vi "CR-导丝颗粒检测1.vi"(8 "error in (no error)":errorcluster caption="错误输入（无错误）", 11 "名称或相对路径":string="Template Program") -> (0 "error in (no error) 2":errorcluster caption="错误输入（无错误）")   [LabVIEW 2017]
uses:
  Picture/SaveButtom.ctl
  Global System.vi
  <vilib>/Utility/xml.llb/Write to XML File(string).vi
panel:
  in  "获取图像":bool
  in  "ROI获取":bool
  in  "创建模板":bool
  in  "保存图像":bool
  out "添加的路径":path
  in  "刷新":bool
  in  "测试按钮":bool
  in  "保存按钮":bool
  in  "Main":enum32{"主参数", "颜色模板匹配参数 ", "测试效果"}(tab)
  in  "导丝颗粒物检测1基础参数":T1={"IsNorImage"=TRUE, "Exposure Values"=100289, "ImagePath"=path "C:/Users/hedongpo/Desktop/514-hdp/Alignment Assemble System/Test Picture/B/3.bmp"} caption="参数界面" {"Exposure Values" scale=0.0..200000.0}
  in  "导丝颗粒物检测1参数":T3={"Rectangle"={"Left"=0, "Top"=0, "Right"=0, "Bottom"=0, "Rotation"=0.0}, "Match Mode "=0, "Minimum Match Score "=800.0, "Number of Matches Requested"=1, "Color Sensitivity "=0, "Color Score Weight "=500.0, "Search Strategy "=0, "Subpixel Accuracy "=FALSE, "Rotation Angle Ranges (degrees)"=[{"Min"=-180.0, "Max"=180.0}], "Match Offset"={"X"=0.0, "Y"=0.0}, "模板路径"=path "C:/Users/delluser001/Desktop/PowerLine Inspect System/Source Code/Template Program/potteryTemplete/Color.png"} {"Search Strategy" items=["Conservative", "Balance", "Aggressive", "Very Aggressive"]; "Color Sensitivity" items=["Low Sensitivity", "Medium Sensitivity", "High Sensitivity"]; "Match Mode" items=["Shift Invariant", "Rotation Invariant"]; "Rectangle"."Rotation" format="%.2f"; "Rectangle"."Left" scale=0.0..1024.0; "Rectangle"."Right" scale=0.0..1024.0}
  out "Number of Features Found":i32
  out "颗粒物有无显示":bool
  in  "Feature Points Strength":string[][](table)
  out "原始图像":T4(plugin-control)
  out "路径输出":path
  in  "Vision Paramter Save Buttom":T5
  out "system time":string
  in  "取消按钮":bool
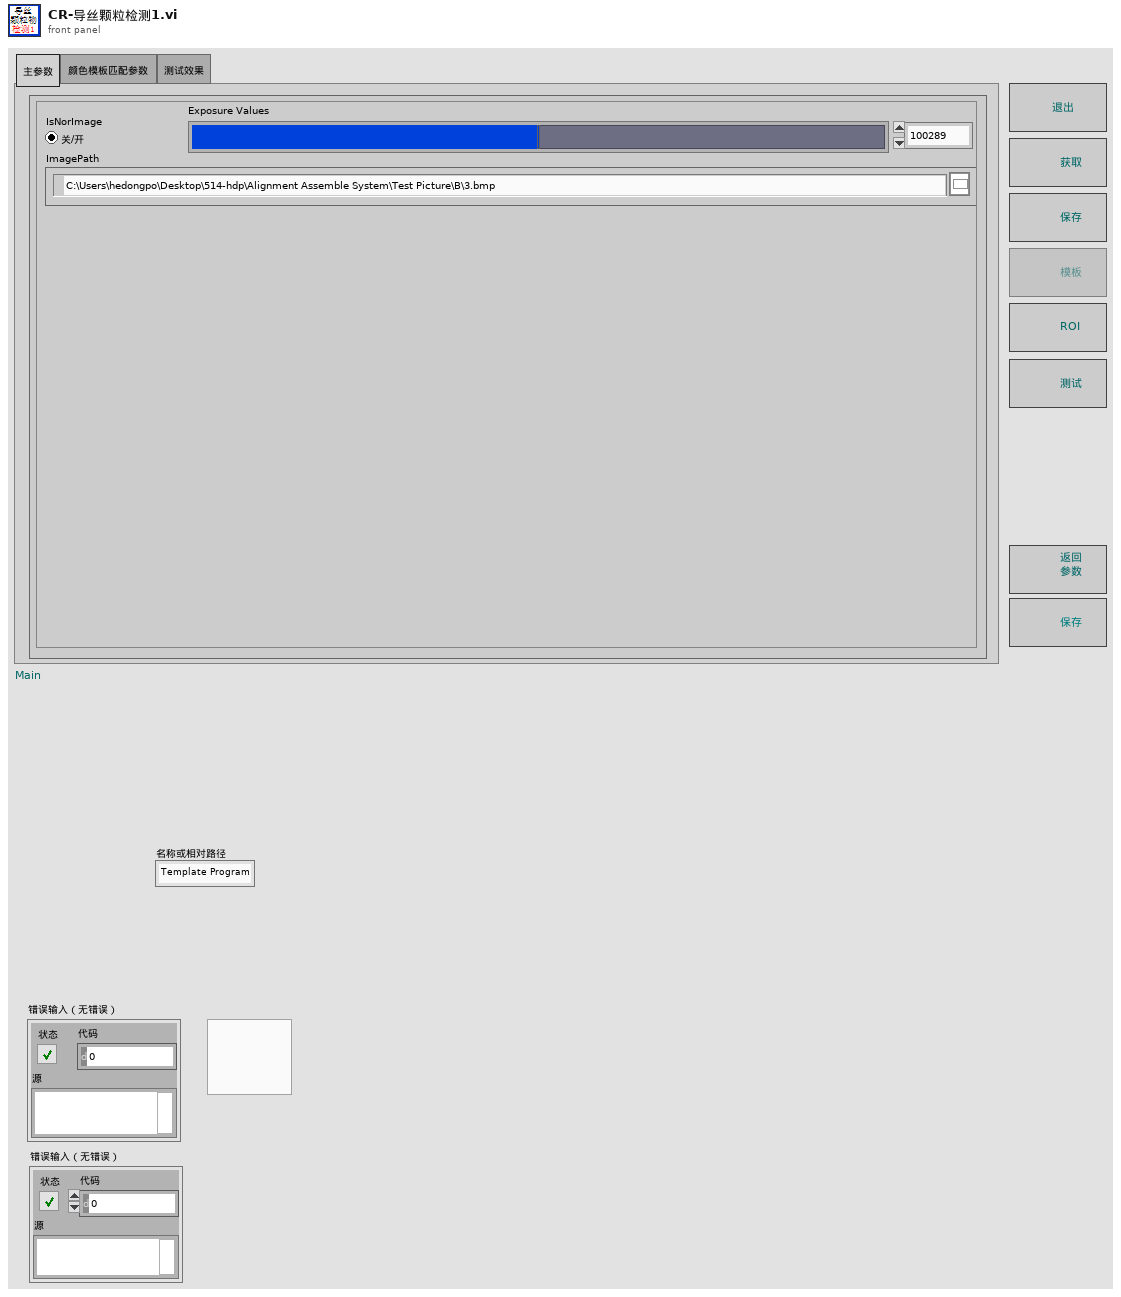
[diagram p1: front panel]
types:
  T1 = cluster{"IsNorImage":bool, "Exposure Values":u32, "ImagePath":path}
  T2 = typedef "IMAQ Rectangle" = cluster{"Left":i32, "Top":i32, "Right":i32, "Bottom":i32, "Rotation":dbl}
  T3 = cluster{"Rectangle":T2, "Match Mode ":u32, "Minimum Match Score ":sgl, "Number of Matches Requested":i32, "Color Sensitivity ":u32, "Color Score Weight ":sgl, "Search Strategy ":u32, "Subpixel Accuracy ":bool, "Rotation Angle Ranges (degrees)":cluster{"Min":sgl, "Max":sgl}[], "Match Offset":cluster{"X":sgl, "Y":sgl}, "模板路径":path}
  T4 = typedef "IMAQ Image.ctl" = refnum<image>
  T5 = typedef "SaveButtom.ctl" = bool
  T6 = cluster{"index":i32, "this vi":refnum<vi>, "error out":errorcluster}
  T7 = cluster{"master data":string, "priority":u16, "secondary data":string[]}
  T8 = cluster{"case name":string[], "queue array":refnum<queue>[]}
  T9 = cluster{"Global Rectangle":i32[], "Contours":cluster{"Contour Type":u32, "ROI Type":u32, "Points":i32[]}[]}
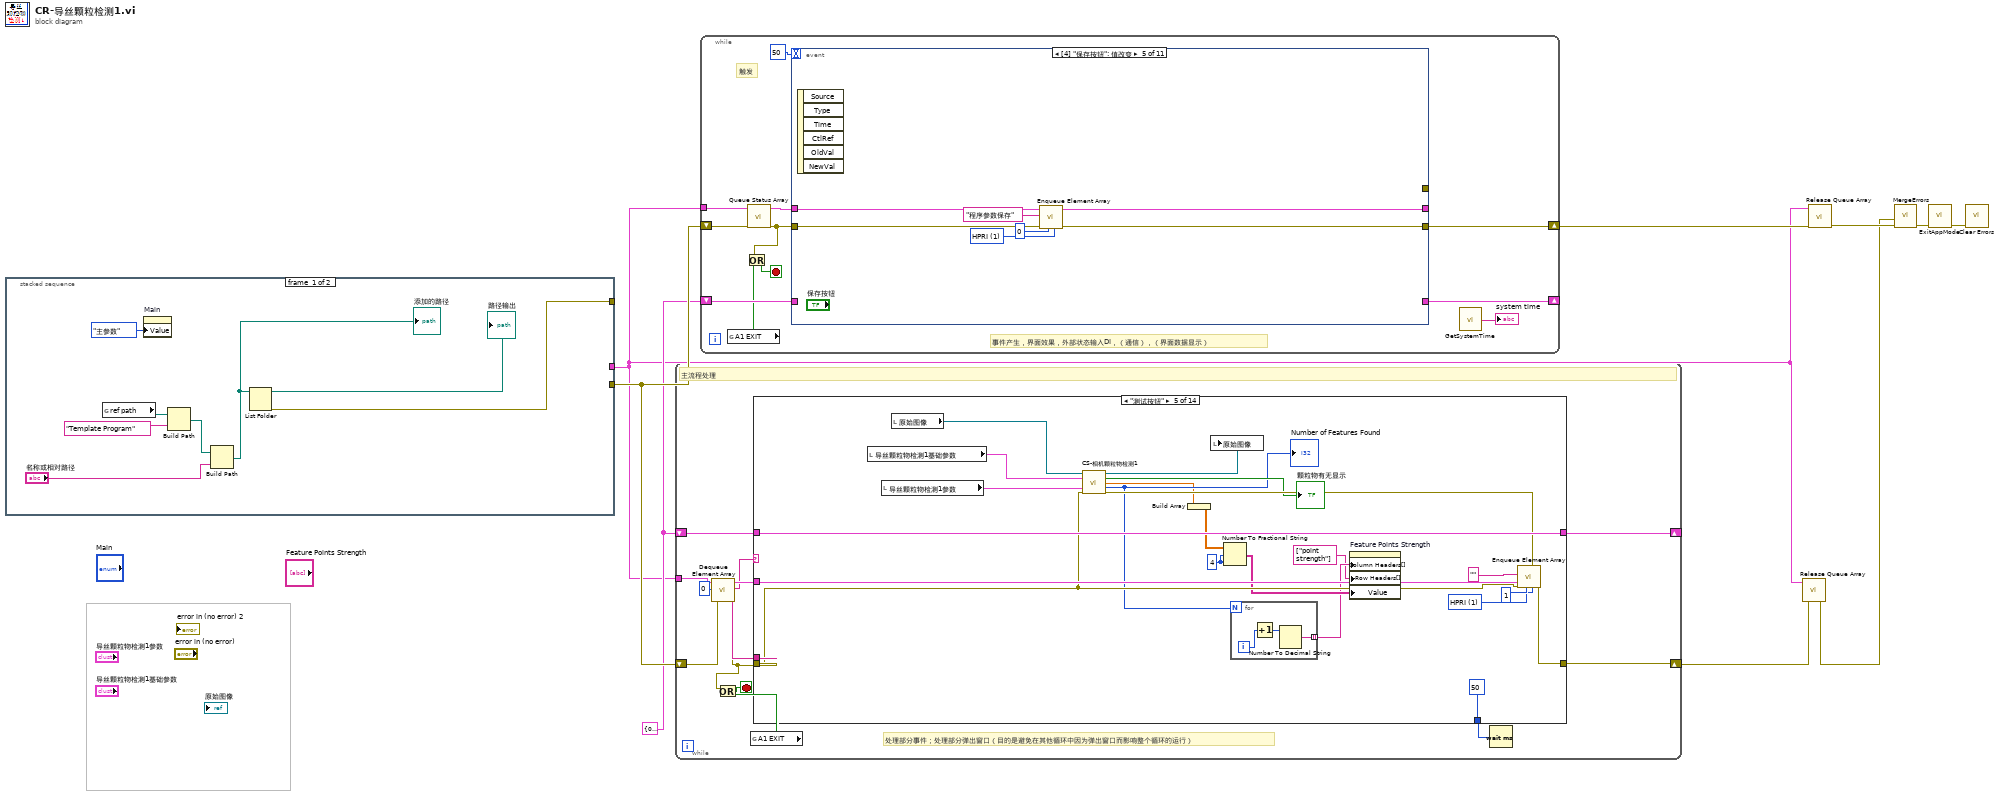
[diagram p0: block diagram]
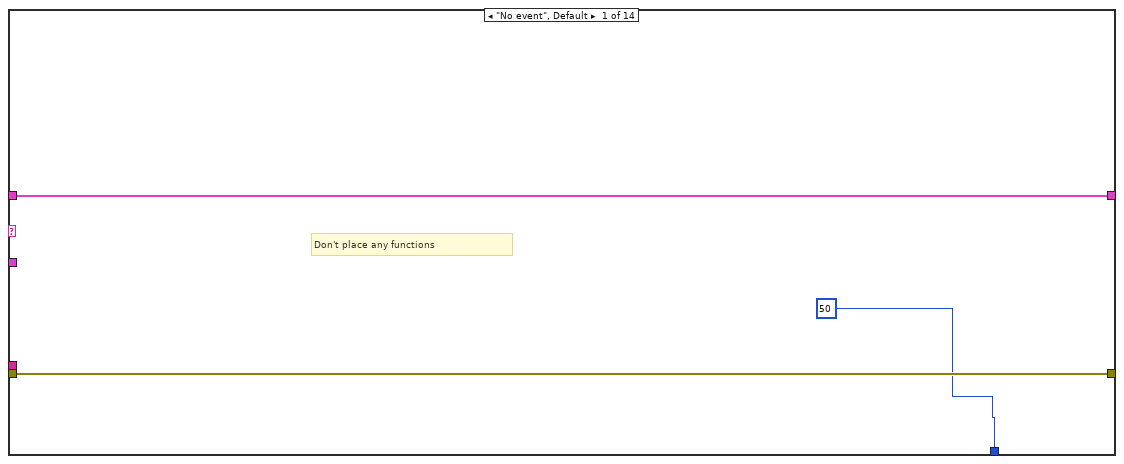
[diagram p2: hidden frame]
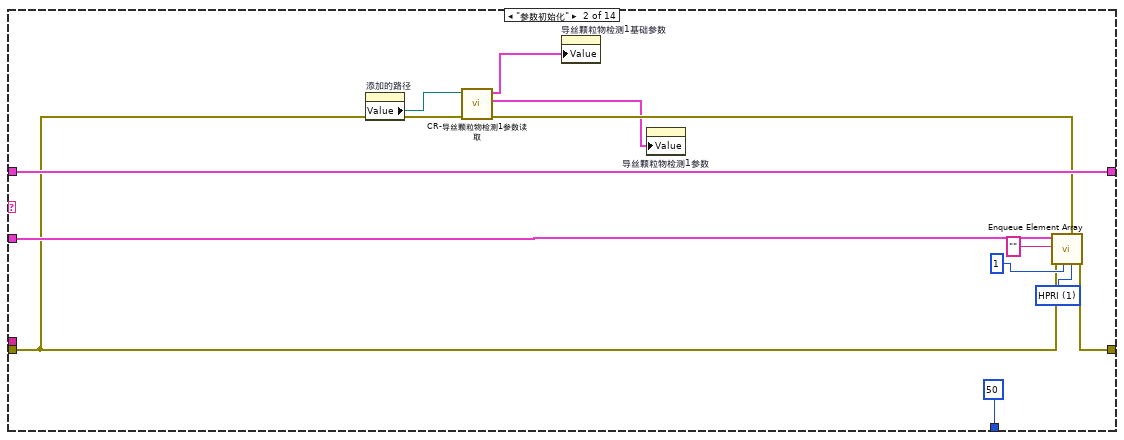
[diagram p3: hidden frame]
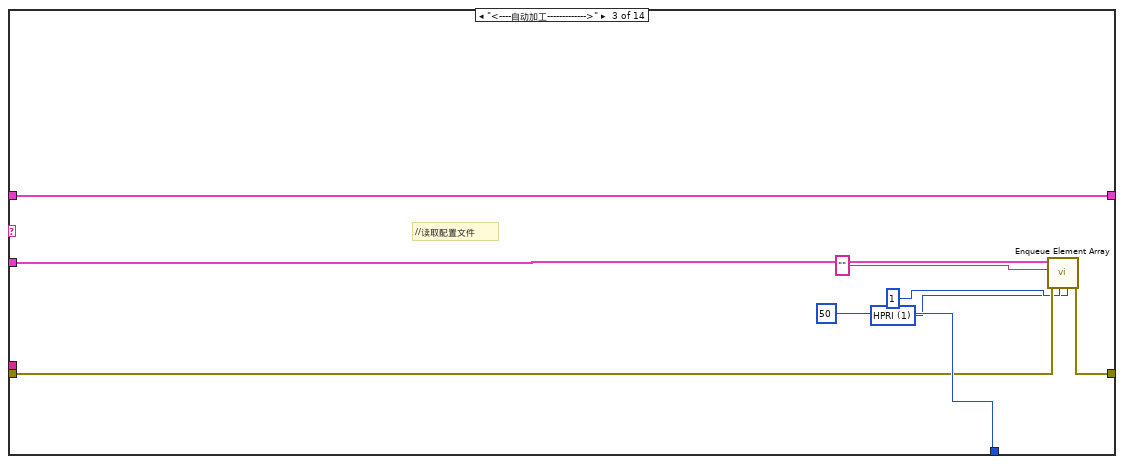
[diagram p4: hidden frame]
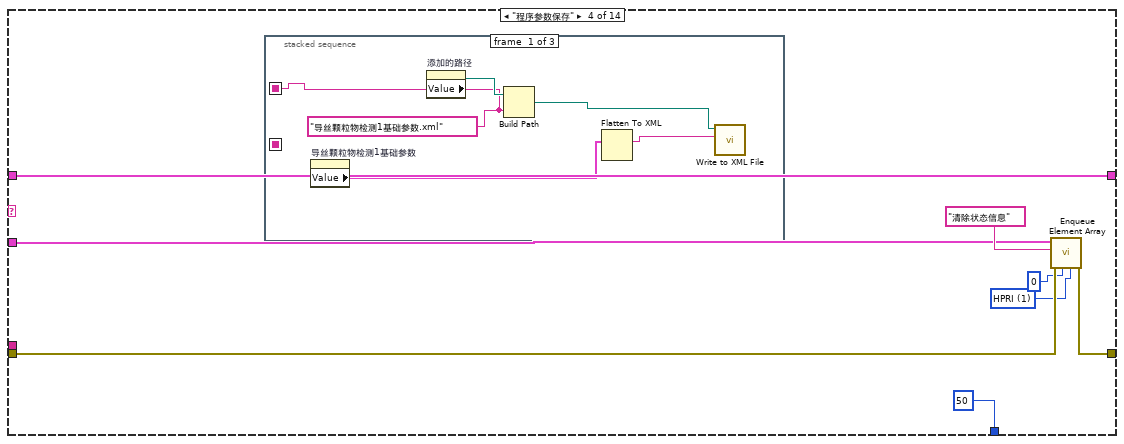
[diagram p5: hidden frame]
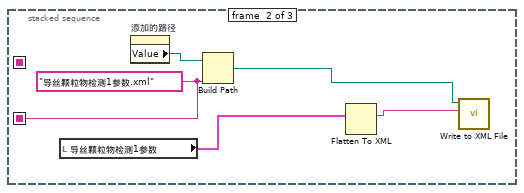
[diagram p6: hidden frame]
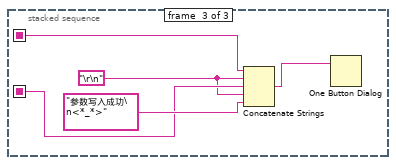
[diagram p7: hidden frame]
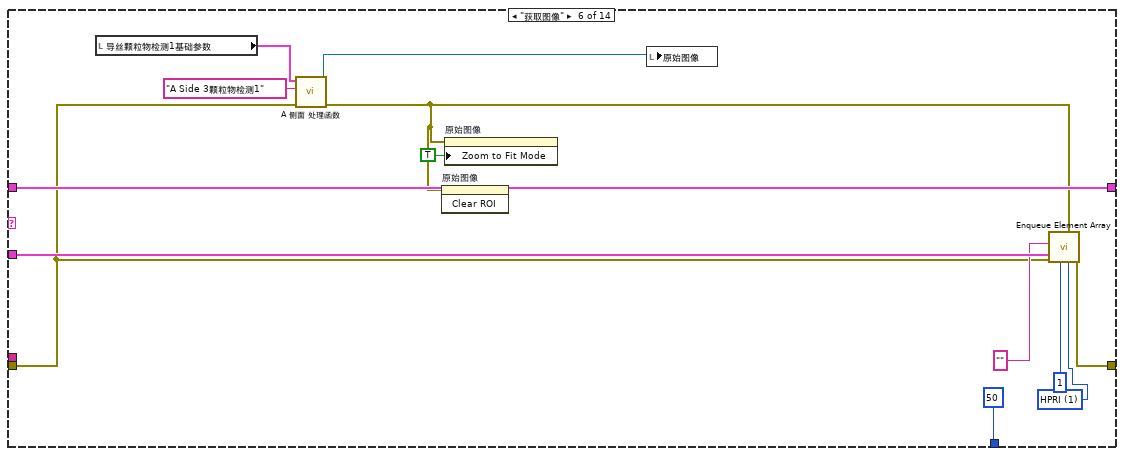
[diagram p8: hidden frame]
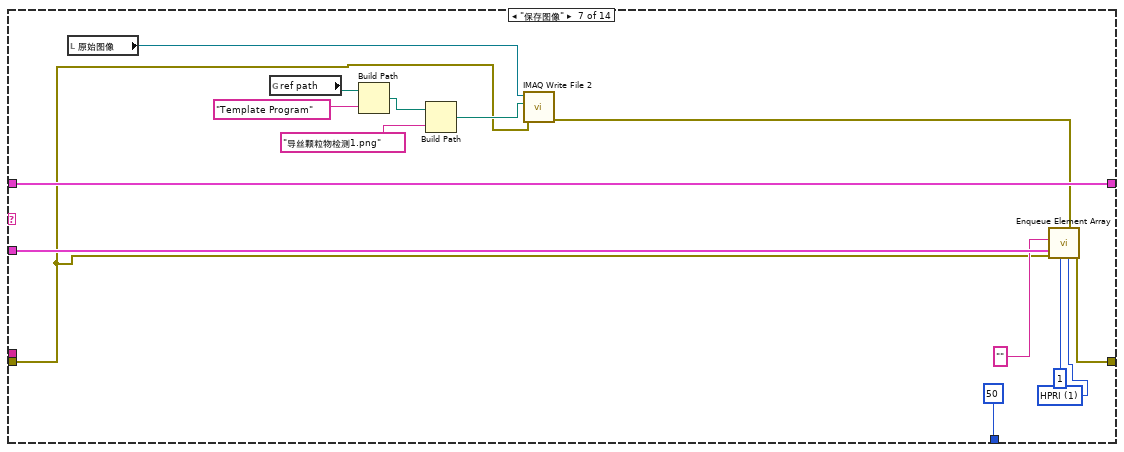
[diagram p9: hidden frame]
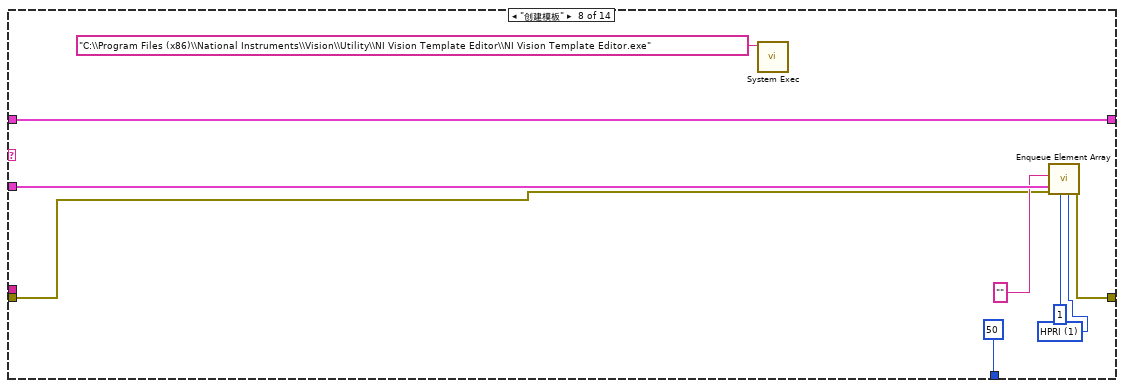
[diagram p10: hidden frame]
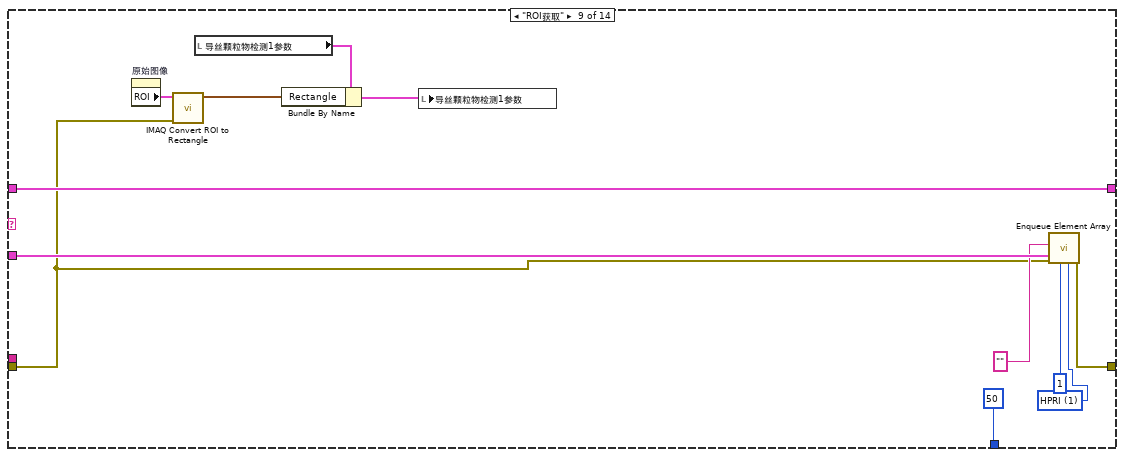
[diagram p11: hidden frame]
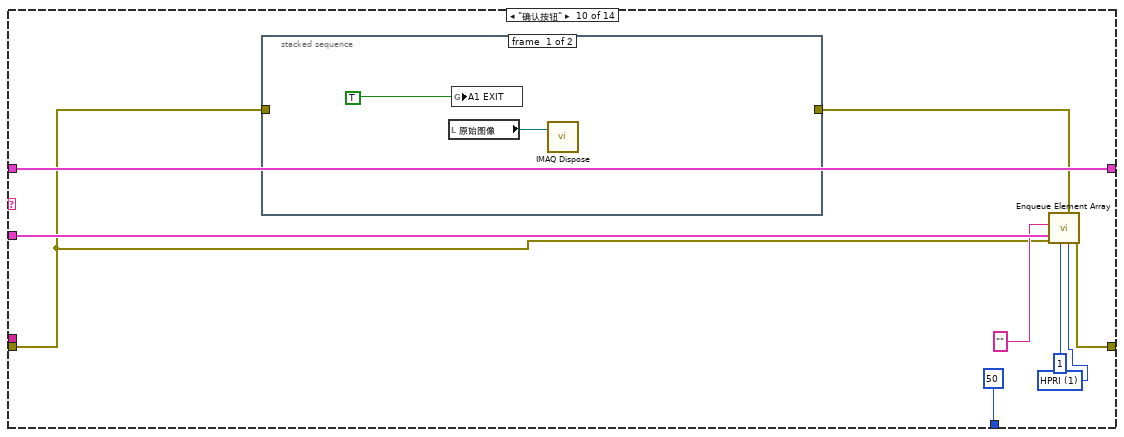
[diagram p12: hidden frame]
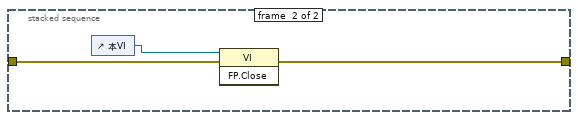
[diagram p13: hidden frame]
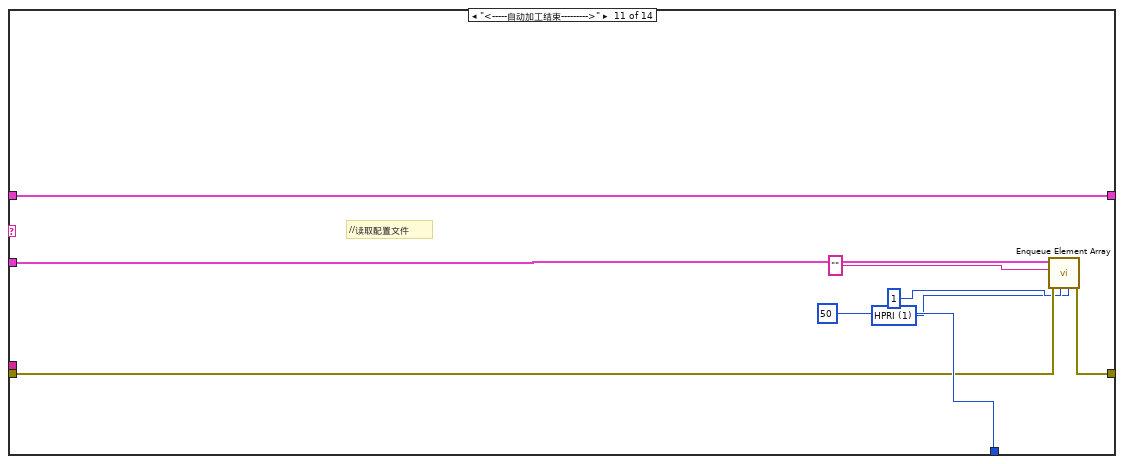
[diagram p14: hidden frame]
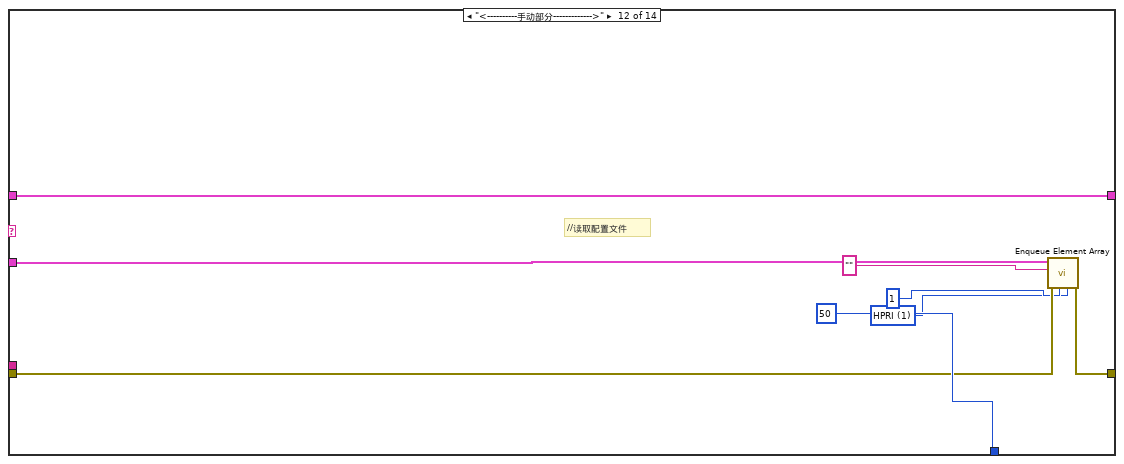
[diagram p15: hidden frame]
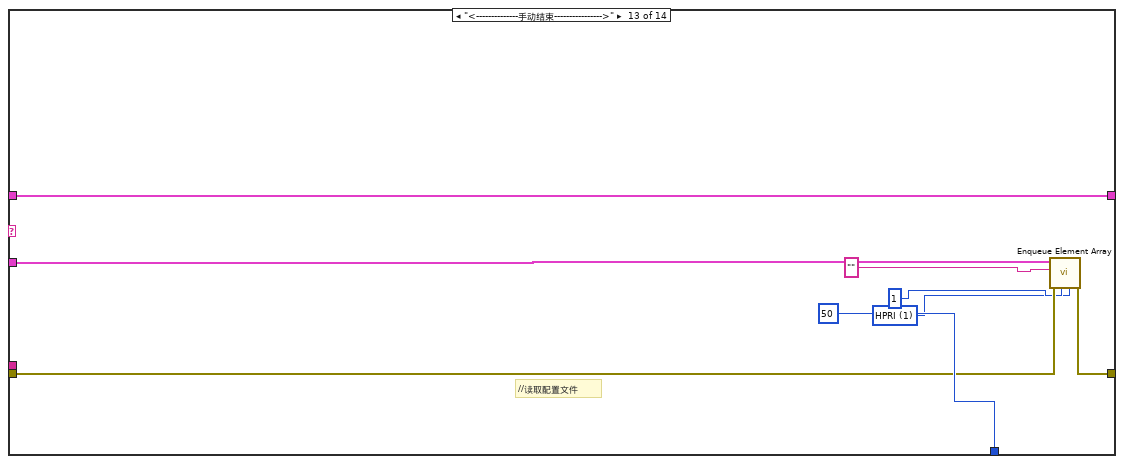
[diagram p16: hidden frame]
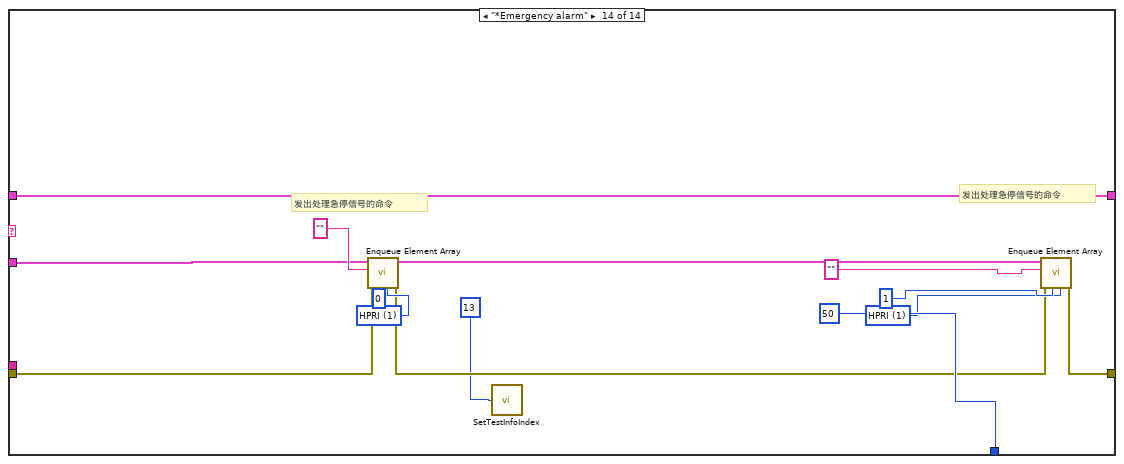
[diagram p17: hidden frame]
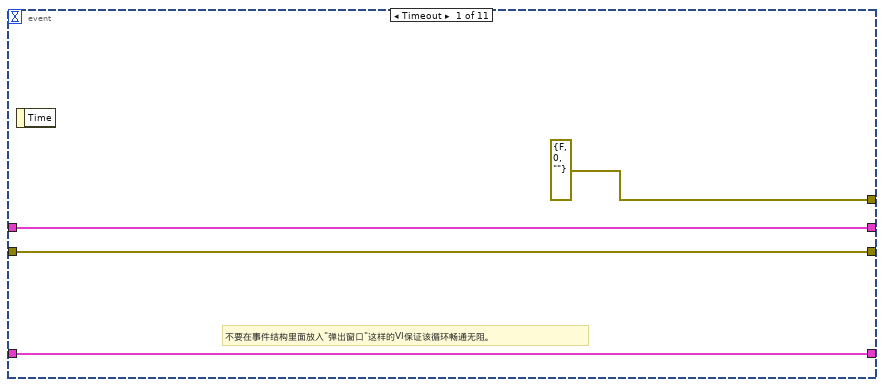
[diagram p18: hidden frame]
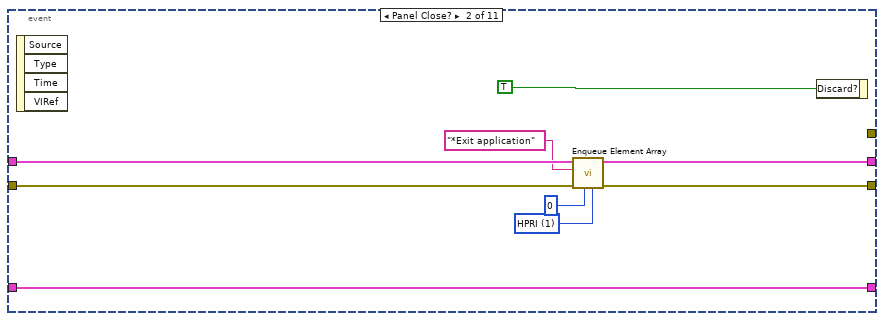
[diagram p19: hidden frame]
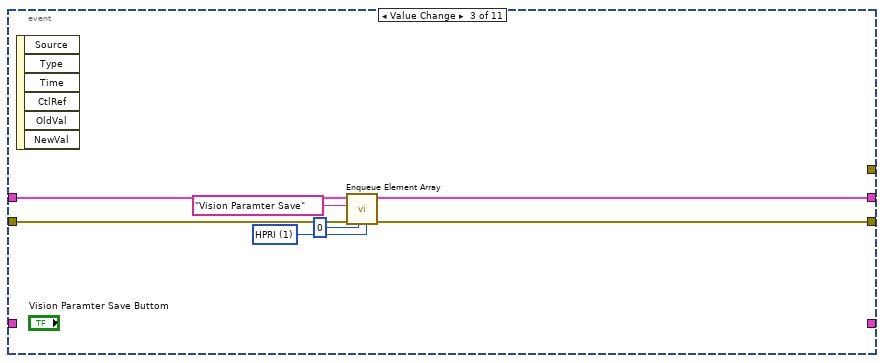
[diagram p20: hidden frame]
diagram:
  w4 = T6 {"index"=0, "this vi"=refnum, "error out"={"status"=FALSE, "code"=0, "source"=""}} ("parameter buffer")
  n1 = stacked-sequence {
    tunnel: [w16 _] -> _
    tunnel: [_ w19] -> w5
    tunnel: [_ w18] -> w1
    frame #0 {
      n2 = global read "Global System.vi" "ref path"() -> (w14:path)
      n3 = property on="Main" class="TabCtl (严格)"("Value"=enum32{"主参数", "颜色模板匹配参数 ", "测试效果"}."主参数" ("Main")) -> ()  [unwired: 2 in, 2 out]
      n4 = Build Path(base path=w14, name or relative path="Template Program" ("名称或相对路径")) -> (appended path=w12:path)
      n5 = Build Path(base path=w12, name or relative path="名称或相对路径") -> (appended path=w10:path)
      "添加的路径" <- w10
      n6 = List Folder(path=w10) -> (path out=→"路径输出":path, error out=w16:errorcluster)  [unwired: 3 in, 2 out]
    }
    frame #1 {
      w27 = string[] ["comm queue1", "data queue 11", "data queue 12", "data queue 13", "data queue 14"]  # queue name
      w28 = 4  # queue num
      w29 = T7 {"master data"="", "priority"=0, "secondary data"=[]}  # element data type
      n7 = call "Obtain Queue Array.vi"("queue name"=w27, "element data type"=w29, "queue num"=w28) -> ("error out"=w23:errorcluster, "queue out"=w24:T8)  [unwired: 2 in, 1 out]
      n8 = call "Enqueue Element Array.vi"("queue index"=0, "error in"=w23, "master data"="参数初始化", "queue in"=w24) -> ("error out"=w22:errorcluster, "queue out"=w21:T8)  [unwired: 6 in]
      n9 = disable-structure shown="启用" {
        disable-tunnel: w22 -> [w35 w36]
        disable-tunnel: w21 -> [w34 w37]
        disable-tunnel: "Loading Variable" ("master data") -> [w33 _]
        disable-tunnel: [w31 w36] -> w19
        disable-tunnel: [w30 w37] -> w18
        frame Disabled {
          n10 = call "Enqueue Element Array.vi"("queue index"=12, "error in"=w35, "master data"=w33, "queue in"=w34) -> ("error out"=w31:errorcluster, "queue out"=w30:T8)  [unwired: 6 in]
        }
        frame Enabled {
        }
      }
    }
  }
  n11 = while {
    shift-right: [w50] -> w3
    shift-left: w5 -> [w41]
    shift-right: [w47] -> _
    shift-left: w4 -> [w48]
    tunnel: w1 -> [w43]
    stop <- w38 stop-if-true
    # "处理部分事件；处理部分弹出窗口（目的是避免在其他循环中因为弹出窗口而影响整个循环的运行）"
    # "主流程处理"
    n12 = call "Dequeue Element Array.vi"("queue in"=w43, "queue index"=0, "error in"=w41) -> ("queue out"=w46:T8, "master data"=w45:string, "secondary data"=w44:string[], "error out"=w40:errorcluster)  [unwired: 2 in, 1 out]
    n13 = global read "Global System.vi" "A1 EXIT"() -> (w39:bool)
    n14 = Or(x=w40, y=w39) -> (x .or. y?=w38:bool)
    n15 = case shown="\"测试按钮\"" w45 {
      tunnel: w46 -> [_ w64 w72 w74 w116 w132 w147 w156 w168 w177 w190 w198 w206 w212]
      tunnel: w40 -> [w52 w57 w68 w78 w109 w123 w134 w150 w161 w171 w186 w194 w202 w209]
      tunnel: [w52 w63 w71 w80 w115 w131 w146 w155 w167 w176 w189 w197 w205 w220] -> w50
      tunnel: [50 50 50 50 50 50 50 50 50 50 50 50 50 50] -> w49
      tunnel: w48 -> [w53 w59 w69 w75 w111 w127 w142 w151 w163 w172 w187 w195 w203 w218]
      tunnel: [w53 w59 w69 w75 w111 w127 w142 w151 w163 w172 w187 w195 w203 w218] -> w47
      tunnel: w44 -> [_ _ _ _ _ _ _ _ _ _ _ _ _ _]
      frame "No event", Default {
        # "Don't place any functions"
      }
      frame "参数初始化" {
        w60 = u16 1 items=["HPRI"=1, "LPRI"=0] ("priority")
        n16 = property on="添加的路径" class="Path"() -> ("Value"=w58:path)  [unwired: 2 in, 2 out]
        n17 = call "CR-导丝颗粒物检测1参数读取.vi"("error in (no error)"=w57, "基路径"=w58) -> ("error out"=w56:errorcluster, "导丝颗粒物检测1参数"=w54:T3, "导丝颗粒物检测1基础参数"=w55:T1)  [unwired: 6 in]
        n18 = property on="导丝颗粒物检测1基础参数" class="Clust (严格)"("Value"=w55) -> ()  [unwired: 2 in, 2 out]
        n19 = property on="导丝颗粒物检测1参数" class="Clust (严格)"("Value"=w54) -> ()  [unwired: 2 in, 2 out]
        n20 = call "Enqueue Element Array.vi"("priority"=w60, "device error in"=w56, "queue index"=1, "error in"=w57, "master data"="" ("Element 1"), "queue in"=w64) -> ("error out"=w63:errorcluster)  [unwired: 4 in, 1 out]
      }
      frame "<----自动加工------------->" {
        w66 = u16 1 items=["HPRI"=1, "LPRI"=0] ("priority")
        # "//读取配置文件"
        n21 = call "Enqueue Element Array.vi"("priority"=w66, "queue index"=1, "error in"=w68, "master data"="" ("Element 1"), "queue in"=w72) -> ("error out"=w71:errorcluster)  [unwired: 5 in, 1 out]
      }
      frame "程序参数保存" {
        w76 = u16 1 items=["HPRI"=1, "LPRI"=0] ("priority")
        n22 = stacked-sequence {
          seq-local: [_ w88 _] -> [_ _ w94]
          seq-local: [w82 _ _] -> [_ _ w92]
          frame #0 {
            w82 = "导丝颗粒物检测1基础参数.xml" ("名称或相对路径")
            n23 = property on="导丝颗粒物检测1基础参数" class="Clust (严格)"() -> ("Value"=w85:T1)  [unwired: 2 in, 2 out]
            n24 = property on="添加的路径" class="Path"() -> ("Value"=w86:path)  [unwired: 2 in, 2 out]
            n25 = Build Path(base path=w86, name or relative path=w82) -> (appended path=w83:path)
            n26 = Flatten To XML(anything=w85) -> (xml string=w84:string)
            n27 = call-poly <vilib>:"Write to XML File.vi"("XML Input"=w84, "XML File Path"=w83) -> ()  [unwired: 7 in, 3 out]
          }
          frame #1 {
            w88 = "导丝颗粒物检测1参数.xml" ("名称或相对路径")
            n28 = local read "导丝颗粒物检测1参数"() -> (w87:T3)
            n29 = property on="添加的路径" class="Path"() -> ("Value"=w91:path)  [unwired: 2 in, 2 out]
            n30 = Build Path(base path=w91, name or relative path=w88) -> (appended path=w89:path)
            n31 = Flatten To XML(anything=w87) -> (xml string=w90:string)
            n32 = call-poly <vilib>:"Write to XML File.vi"("XML Input"=w90, "XML File Path"=w89) -> ()  [unwired: 7 in, 3 out]
          }
          frame #2 {
            w93 = "\r\n"
            n33 = Concatenate Strings(w92, w93, w94, w93, "参数写入成功\n<*_*>" ("消息")) -> (w95:string)
            n34 = One Button Dialog(message=w95) -> ()  [unwired: 1 in, 1 out]
          }
        }
        n35 = call "Enqueue Element Array.vi"("priority"=w76, "queue index"=0, "error in"=w78, "master data"="清除状态信息" ("Element 1"), "queue in"=w74) -> ("error out"=w80:errorcluster)  [unwired: 5 in, 1 out]
      }
      frame "测试按钮" {
        w101 = i16 4 ("精度(6)")
        w112 = u16 1 items=["HPRI"=1, "LPRI"=0] ("priority")
        n36 = local read "导丝颗粒物检测1基础参数"() -> (w110:T1)
        n37 = local read "导丝颗粒物检测1参数"() -> (w105:T3)
        n38 = local read "原始图像"() -> (w107:T4)
        n39 = call "CS-相机颗粒物检测1.vi"("Image in"=w107, "相机颗粒物检测1基础参数"=w110, "相机颗粒物检测1参数"=w105, "error in (no error)"=w109) -> ("Image out"=w108:T4, "颗粒物有无显示"=→"颗粒物有无显示":bool, "颗粒物大小显示"=w102:dbl[], "Number of Features Found"=w103:i32, "error out"=w106:errorcluster)  [unwired: 6 in, 1 out]
        "Number of Features Found" <- w103
        n40 = Build Array(w102) -> (w100:dbl[][])
        n41 = local write "原始图像"(w108) -> ()
        n42 = Number To Fractional String(number=w100, width (-)=w101, precision (6)=w101) -> (F-format string=w99:string[][])  [unwired: 1 in]
        n43 = for {
          N: w103 -> [_]
          tunnel: [w118] -> w98 mode=indexing
          i -> [w120]
          n44 = Increment(x=w120) -> (x+1=w119:i32)
          n45 = Number To Decimal String(number=w119) -> (decimal integer string=w118:string)  [unwired: 1 in]
        }
        n46 = property on="Feature Points Strength" class="Tbl (严格)"("Column Headers[]"=w98, "Row Headers[]"=string[] ["point strength"] ("列首字符串[]"), "Value"=w99) -> ()  [unwired: 2 in, 2 out]
        n47 = call "Enqueue Element Array.vi"("priority"=w112, "device error in"=w106, "queue index"=1, "error in"=w109, "master data"="" ("Element 1"), "queue in"=w116) -> ("error out"=w115:errorcluster)  [unwired: 4 in, 1 out]
      }
      frame "获取图像" {
        w128 = u16 1 items=["HPRI"=1, "LPRI"=0] ("priority")
        n48 = local read "导丝颗粒物检测1基础参数"() -> (w125:T1)
        n49 = call "A 侧面 处理函数.vi"("error in (no error)"=w123, "Image Name"="A Side 3颗粒物检测1", "ParamsUI"=w125) -> ("error out"=w121:errorcluster, "Image out"=w124:T4)  [unwired: 5 in, 2 out]
        n50 = invoke on="原始图像" class="ImageControl" method="Clear ROI"(error in=w121) -> ()  [unwired: 2 in, 3 out]
        n51 = property on="原始图像" class="ImageControl"(error in=w121, "Zoom to Fit Mode"=TRUE) -> ()  [unwired: 1 in, 2 out]
        n52 = local write "原始图像"(w124) -> ()
        n53 = call "Enqueue Element Array.vi"("priority"=w128, "device error in"=w121, "queue index"=1, "error in"=w123, "master data"="" ("Element 1"), "queue in"=w132) -> ("error out"=w131:errorcluster)  [unwired: 4 in, 1 out]
      }
      frame "保存图像" {
        w143 = u16 1 items=["HPRI"=1, "LPRI"=0] ("priority")
        n54 = local read "原始图像"() -> (w135:T4)
        n55 = global read "Global System.vi" "ref path"() -> (w141:path)
        n56 = Build Path(base path=w141, name or relative path="Template Program" ("名称或相对路径")) -> (appended path=w139:path)
        n57 = Build Path(base path=w139, name or relative path="导丝颗粒物检测1.png" ("名称或相对路径")) -> (appended path=w137:path)
        n58 = call-poly "IMAQ Write File 2"("error in (no error)"=w134, "File Path"=w137, "Image"=w135) -> ("error out"=w136:errorcluster)  [unwired: 7 in, 1 out]
        n59 = call "Enqueue Element Array.vi"("priority"=w143, "device error in"=w136, "queue index"=1, "error in"=w134, "master data"="" ("Element 1"), "queue in"=w147) -> ("error out"=w146:errorcluster)  [unwired: 4 in, 1 out]
      }
      frame "创建模板" {
        w152 = u16 1 items=["HPRI"=1, "LPRI"=0] ("priority")
        n60 = call <vilib>:"System Exec.vi"("command line"="C:\\Program Files (x86)\\National Instruments\\Vision\\Utility\\NI Vision Template Editor\\NI Vision Template Editor.exe") -> ()  [unwired: 7 in, 4 out]
        n61 = call "Enqueue Element Array.vi"("priority"=w152, "queue index"=1, "error in"=w150, "master data"="" ("Element 1"), "queue in"=w156) -> ("error out"=w155:errorcluster)  [unwired: 5 in, 1 out]
      }
      frame "ROI获取" {
        w164 = u16 1 items=["HPRI"=1, "LPRI"=0] ("priority")
        n62 = property on="原始图像" class="ImageControl"() -> ("ROI"=w162:T9)  [unwired: 2 in, 2 out]
        n63 = call "IMAQ Convert ROI to Rectangle"("error in (no error)"=w161, "ROI Descriptor"=w162) -> ("Rectangle"=w159:T2)  [unwired: 7 in, 1 out]
        n64 = local read "导丝颗粒物检测1参数"() -> (w160:T3)
        n65 = Bundle By Name(cluster=w160, "Rectangle"=w159) -> (w158:T3)
        n66 = local write "导丝颗粒物检测1参数"(w158) -> ()
        n67 = call "Enqueue Element Array.vi"("priority"=w164, "queue index"=1, "error in"=w161, "master data"="" ("Element 1"), "queue in"=w168) -> ("error out"=w167:errorcluster)  [unwired: 5 in, 1 out]
      }
      frame "确认按钮" {
        w173 = u16 1 items=["HPRI"=1, "LPRI"=0] ("priority")
        n68 = stacked-sequence {
          tunnel: w171 -> [_ w182]
          tunnel: [_ w181] -> w170
          frame #0 {
            n69 = local read "原始图像"() -> (w179:T4)
            n70 = global write "Global System.vi" "A1 EXIT"(TRUE ("EXIT")) -> ()
            n71 = call "IMAQ Dispose"("Image"=w179) -> ()  [unwired: 5 in, 1 out]
          }
          frame #1 {
            n72 = control-ref of="本VI"() -> (w183:refnum<vi>)
            n73 = invoke class="VI" method="FP.Close"(reference=w183, error in=w182) -> (error out=w181:errorcluster)  [unwired: 1 in, 2 out]
          }
        }
        n74 = call "Enqueue Element Array.vi"("priority"=w173, "device error in"=w170, "queue index"=1, "error in"=w171, "master data"="" ("Element 1"), "queue in"=w177) -> ("error out"=w176:errorcluster)  [unwired: 4 in, 1 out]
      }
      frame "<-----自动加工结束--------->" {
        w184 = u16 1 items=["HPRI"=1, "LPRI"=0] ("priority")
        # "//读取配置文件"
        n75 = call "Enqueue Element Array.vi"("priority"=w184, "queue index"=1, "error in"=w186, "master data"="" ("Element 1"), "queue in"=w190) -> ("error out"=w189:errorcluster)  [unwired: 5 in, 1 out]
      }
      frame "<----------手动部分------------->" {
        w192 = u16 1 items=["HPRI"=1, "LPRI"=0] ("priority")
        # "//读取配置文件"
        n76 = call "Enqueue Element Array.vi"("priority"=w192, "queue index"=1, "error in"=w194, "master data"="" ("Element 1"), "queue in"=w198) -> ("error out"=w197:errorcluster)  [unwired: 5 in, 1 out]
      }
      frame "<--------------手动结束---------------->" {
        w200 = u16 1 items=["HPRI"=1, "LPRI"=0] ("priority")
        # "//读取配置文件"
        n77 = call "Enqueue Element Array.vi"("priority"=w200, "queue index"=1, "error in"=w202, "master data"="" ("Element 1"), "queue in"=w206) -> ("error out"=w205:errorcluster)  [unwired: 5 in, 1 out]
      }
      frame "*Emergency alarm" {
        w215 = u16 1 items=["HPRI"=1, "LPRI"=0] ("priority")
        w216 = u16 1 items=["HPRI"=1, "LPRI"=0] ("priority")
        # "发出处理急停信号的命令"
        # "发出处理急停信号的命令"
        n78 = call "Enqueue Element Array.vi"("priority"=w215, "queue index"=0, "error in"=w209, "master data"="" ("Element 1"), "queue in"=w212) -> ("error out"=w210:errorcluster, "queue out"=w211:T8)  [unwired: 5 in]
        n79 = call "SetTestInfoIndex.vi"("test info index"=13) -> ()
        n80 = call "Enqueue Element Array.vi"("priority"=w216, "queue index"=1, "error in"=w210, "master data"="" ("Element 1"), "queue in"=w211) -> ("error out"=w220:errorcluster)  [unwired: 5 in, 1 out]
      }
    }
    n81 = Wait (ms)(milliseconds to wait=w49) -> ()  [unwired: 1 out]
  }
  n82 = while {
    shift-right: [w225] -> w6
    shift-left: w5 -> [w229]
    shift-right: [w227] -> _
    shift-left: w4 -> [w228]
    tunnel: w1 -> [w231]
    stop <- w222 stop-if-true
    # "触发"
    # "事件产生，界面效果，外部状态输入DI，（通信），（界面数据显示）"
    n83 = global read "Global System.vi" "A1 EXIT"() -> (w223:bool)
    n84 = call "Queue Status Array.vi"("error in (no error)"=w229, "queue in"=w231) -> ("error out"=w224:errorcluster, "queue out"=w226:T8)  [unwired: 4 in]
    n85 = Or(x=w224, y=w223) -> (x .or. y?=w222:bool)
    n86 = event shown="[4] \"保存按钮\": 值改变" {
      selector: _ -> [_ _ _ _ _ _ _ _ _ _ _]
      dyn-events: _ -> [_ _ _ _ _ _ _ _ _ _ _]
      timeout: 50 -> [_ _ _ _ _ _ _ _ _ _ _]
      tunnel: w228 -> [w236 w244 _ _ _ _ _ _ _ _ _]
      tunnel: [w236 w244 _ _ _ _ _ _ _ _ _] -> w227
      tunnel: [errorcluster {"status"=FALSE, "code"=0, "source"=""} ("error out") _ _ _ _ _ _ _ _ _ _] -> _
      tunnel: w226 -> [w234 w243 w249 w256 w263 w271 w278 w285 w293 w301 w309]
      tunnel: w224 -> [w233 w242 w248 w255 w262 w270 w277 w284 w292 w300 w308]
      tunnel: [w233 w241 w246 w253 w260 w268 w275 w282 w290 w298 w306] -> w225
      tunnel: [w234 w240 w247 w254 w261 w269 w276 w283 w291 w299 w307] -> _
      event Timeout {
        # "不要在事件结构里面放入\"弹出窗口\"这样的VI保证该循环畅通无阻。"
        n87 = event-data() -> ()  [unwired: 1 in, 1 out]
      }
      event Panel Close? {
        w238 = u16 1 items=["HPRI"=1, "LPRI"=0] ("priority")
        n88 = event-data() -> ()  [unwired: 1 in, 4 out]
        n89 = call "Enqueue Element Array.vi"("priority"=w238, "queue index"=0, "error in"=w242, "master data"="*Exit application", "queue in"=w243) -> ("error out"=w241:errorcluster, "queue out"=w240:T8)  [unwired: 5 in]
        n90 = event-data("Discard?"=TRUE) -> ()  [unwired: 1 in, 1 out]
      }
      event Value Change {
        w251 = u16 1 items=["HPRI"=1, "LPRI"=0] ("priority")
        n91 = event-data() -> ()  [unwired: 1 in, 6 out]
        n92 = call "Enqueue Element Array.vi"("priority"=w251, "queue index"=0, "error in"=w248, "master data"="Vision Paramter Save", "queue in"=w249) -> ("error out"=w246:errorcluster, "queue out"=w247:T8)  [unwired: 5 in]
      }
      event "取消按钮": Value Change {
        w258 = u16 1 items=["HPRI"=1, "LPRI"=0] ("priority")
        n93 = event-data() -> ()  [unwired: 1 in, 6 out]
        n94 = call "Enqueue Element Array.vi"("priority"=w258, "queue index"=0, "error in"=w255, "master data"="确认按钮", "queue in"=w256) -> ("error out"=w253:errorcluster, "queue out"=w254:T8)  [unwired: 5 in]
      }
      event "保存按钮": Value Change {
        w265 = u16 1 items=["HPRI"=1, "LPRI"=0] ("priority")
        n95 = event-data() -> ()  [unwired: 1 in, 6 out]
        n96 = call "Enqueue Element Array.vi"("priority"=w265, "queue index"=0, "error in"=w262, "master data"="程序参数保存", "queue in"=w263) -> ("error out"=w260:errorcluster, "queue out"=w261:T8)  [unwired: 5 in]
      }
      event "获取图像": Value Change {
        w273 = u16 1 items=["HPRI"=1, "LPRI"=0] ("priority")
        n97 = event-data() -> ()  [unwired: 1 in, 6 out]
        n98 = property on="Main" class="TabCtl (严格)"("Value"=enum32{"主参数", "颜色模板匹配参数 ", "测试效果"}."测试效果" ("Main")) -> ()  [unwired: 2 in, 2 out]
        n99 = call "Enqueue Element Array.vi"("priority"=w273, "queue index"=0, "error in"=w270, "master data"="获取图像", "queue in"=w271) -> ("error out"=w268:errorcluster, "queue out"=w269:T8)  [unwired: 5 in]
      }
      event "保存图像": Value Change {
        w280 = u16 1 items=["HPRI"=1, "LPRI"=0] ("priority")
        n100 = event-data() -> ()  [unwired: 1 in, 6 out]
        n101 = call "Enqueue Element Array.vi"("priority"=w280, "queue index"=0, "error in"=w277, "master data"="保存图像", "queue in"=w278) -> ("error out"=w275:errorcluster, "queue out"=w276:T8)  [unwired: 5 in]
      }
      event "创建模板": Value Change {
        w287 = u16 1 items=["HPRI"=1, "LPRI"=0] ("priority")
        n102 = event-data() -> ()  [unwired: 1 in, 6 out]
        n103 = call "Enqueue Element Array.vi"("priority"=w287, "queue index"=0, "error in"=w284, "master data"="创建模板", "queue in"=w285) -> ("error out"=w282:errorcluster, "queue out"=w283:T8)  [unwired: 5 in]
      }
      event "ROI获取": Value Change {
        w295 = u16 1 items=["HPRI"=1, "LPRI"=0] ("priority")
        n104 = event-data() -> ()  [unwired: 1 in, 6 out]
        n105 = property on="Main" class="TabCtl (严格)"("Value"=enum32{"主参数", "颜色模板匹配参数 ", "测试效果"}."颜色模板匹配参数 " ("Main")) -> ()  [unwired: 2 in, 2 out]
        n106 = call "Enqueue Element Array.vi"("priority"=w295, "queue index"=0, "error in"=w292, "master data"="ROI获取", "queue in"=w293) -> ("error out"=w290:errorcluster, "queue out"=w291:T8)  [unwired: 5 in]
      }
      event "测试按钮": Value Change {
        w303 = u16 1 items=["HPRI"=1, "LPRI"=0] ("priority")
        n107 = event-data() -> ()  [unwired: 1 in, 6 out]
        n108 = property on="Main" class="TabCtl (严格)"("Value"=enum32{"主参数", "颜色模板匹配参数 ", "测试效果"}."测试效果" ("Main")) -> ()  [unwired: 2 in, 2 out]
        n109 = call "Enqueue Element Array.vi"("priority"=w303, "queue index"=0, "error in"=w300, "master data"="测试按钮", "queue in"=w301) -> ("error out"=w298:errorcluster, "queue out"=w299:T8)  [unwired: 5 in]
      }
      event "刷新": Value Change {
        n110 = event-data() -> ()  [unwired: 1 in, 6 out]
        n111 = disable-structure shown="禁用" {
          disable-tunnel: w309 -> [w313 _]
          disable-tunnel: w308 -> [w312 _]
          disable-tunnel: [w311 _] -> w307
          disable-tunnel: [w310 _] -> w306
          frame Disabled {
            w315 = u16 1 items=["HPRI"=1, "LPRI"=0] ("priority")
            # "刷新"
            n112 = call "Enqueue Element Array.vi"("priority"=w315, "queue index"=0, "error in"=w312, "master data"="刷新", "queue in"=w313) -> ("error out"=w310:errorcluster, "queue out"=w311:T8)  [unwired: 5 in]
          }
          frame Enabled {
          }
        }
        n113 = property on="Main" class="TabCtl (严格)"("Value"=enum32{"主参数", "颜色模板匹配参数 ", "测试效果"}."颜色模板匹配参数 " ("Main")) -> ()  [unwired: 2 in, 2 out]
      }
    }
    n114 = call "GetSystemTime.vi"() -> ("date/time string"=→"system time":string)  [unwired: 7 in]
  }
  n115 = call "Release Queue Array.vi"("error in"=w3, "queue in"=w1) -> ("error out"=w2:errorcluster)  [unwired: 2 in, 3 out]
  n116 = call "Release Queue Array.vi"("error in"=w6, "queue in"=w1) -> ("error out"=w9:errorcluster)  [unwired: 2 in, 3 out]
  n117 = call "MergeErrors.vi"("error in 3 (no error)"=w2, "error in 4 (no error)"=w9) -> ("error out"=w8:errorcluster)  [unwired: 6 in]
  n118 = call "ExitAppMode.vi"("error in (no error)"=w8) -> ("error out"=w7:errorcluster)  [unwired: 10 in]
  n119 = call <vilib>:"Clear Errors.vi"("error in (no error)"=w7) -> ()  [unwired: 5 in, 2 out]
